vi "4461 - Create Tasks AI.vi"(8 "error in (no error)":errorcluster, 11 "Instrument.Lockin in":refnum<class "Instrument.Lockin.lvclass">) -> (0 "error out":errorcluster, 3 "Instrument.Lockin out":refnum<class "Instrument.Lockin.lvclass">)   [LabVIEW 2016, in "LockinDAQ.lvclass"]
uses:
  LockinDAQ.lvclass
  <resource>/objmgr/daqmx.rc
  <vilib>/DAQmx/create/channels.llb/DAQmx Create Channel (AI-Voltage-Basic).vi
  Instrument.Lockin/Instrument.Lockin.lvclass
  C:/Program Files (x86)/National Instruments/LabVIEW 2016/user.lib/LevyLab/Levylab Instruments/SMOs/Instrument/Instrument.lvclass
  C:/Program Files (x86)/National Instruments/LabVIEW 2016/user.lib/LevyLab/Levylab Instruments/SMOs/LevyLab/LevyLab.lvclass
  C:/Program Files (x86)/National Instruments/LabVIEW 2016/vi.lib/JKI/JKI SMO/SMO/SMO.lvclass
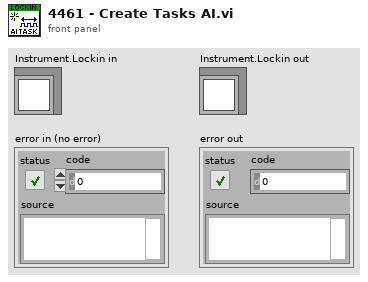
[diagram p1: front panel]
types:
  T1 = typedef "LockinDAQ.lvclass/DAQType-enum.ctl" = enum16{"None", "USB 4431", "PXI 446x"}
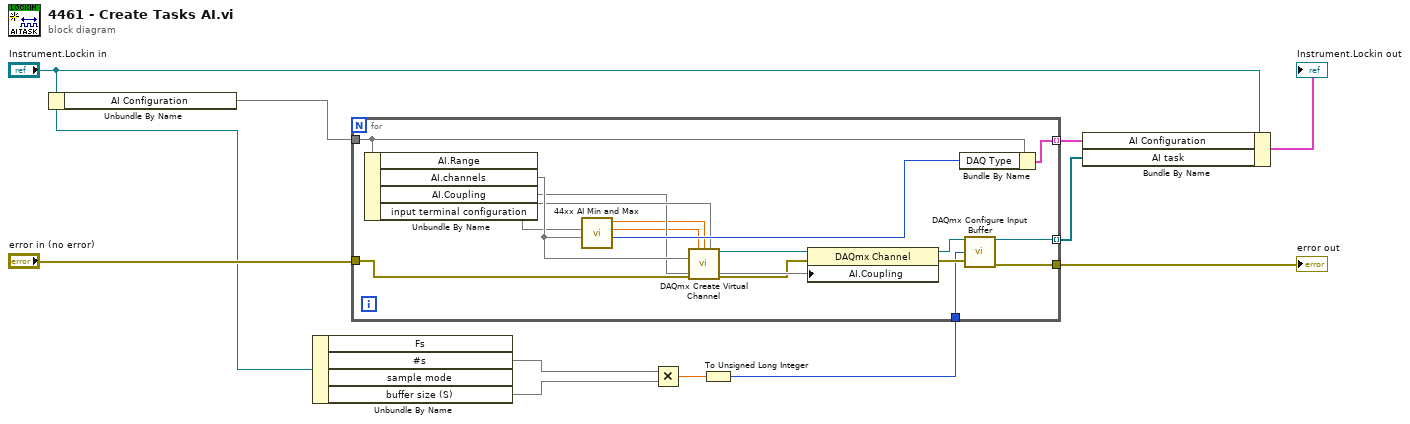
[diagram p0: block diagram]
diagram:
  n1 = Unbundle By Name("Instrument.Lockin in") -> ("AI Configuration"=w8)
  n2 = Unbundle By Name("Instrument.Lockin in") -> ("#s"=w6, "buffer size (S)"=w5)  [unwired: 2 out]
  n3 = Multiply(x=w6, y=w5) -> (x*y=w7:dbl)
  n4 = To Unsigned Long Integer(number=w7) -> (unsigned 32bit integer=w4:u32)
  n5 = for {
    tunnel: [w13] -> w2 mode=indexing
    tunnel: w8 -> [w18]
    tunnel: "error in (no error)" -> [w19]
    tunnel: [w16] -> w10
    tunnel: w4 -> [w14]
    tunnel: [w12] -> w1 mode=indexing
    n6 = Unbundle By Name(w18) -> ("AI.Range"=w24, "AI.channels"=w28, "AI.Coupling"=w25, "input terminal configuration"=w26)
    n7 = call "44xx AI Min and Max.vi"("AI.channels"=w28, "446x AI"=w24) -> ("DAQ Type"=w27:T1, "AI.Max"=w22:dbl, "AI.Min"=w23:dbl)  [unwired: 7 in]
    n8 = call-poly <vilib>:"DAQmx Create Virtual Channel.vi"("maximum value"=w22, "minimum value"=w23, "input terminal configuration"=w26, "physical channels"=w28, "error in"=w19) -> ("task out"=w20:refnum<k21>, "error out"=w21:errorcluster)  [unwired: 9 in]
    n9 = property class="DAQmx Channel"(reference=w20, error in=w21, "AI.Coupling"=w25) -> (reference out=w15:refnum<k21>, error out=w17:errorcluster)
    n10 = Bundle By Name(cluster=w18, "DAQ Type"=w27) -> (w13:cluster{})
    n11 = call <vilib>:"DAQmx Configure Input Buffer.vi"("task/channels in"=w15, "buffer size (in samples per channel)"=w14, "error in"=w17) -> ("task out"=w12:refnum<k21>, "error out"=w16:errorcluster)  [unwired: 11 in]
  }
  "error out" <- w10
  n12 = Bundle By Name(cluster="Instrument.Lockin in", "AI Configuration"=w2, "AI task"=w1) -> (→"Instrument.Lockin out":cluster{})
